vi "Write File Path.vi"(8 "error in (no error)":errorcluster, 10 "File Path":path, 11 "File Parser Interface in":refnum<class "File Parser Interface.lvclass">) -> (0 "error out":errorcluster, 3 "File Parser Interface out":refnum<class "File Parser Interface.lvclass">)   [LabVIEW 2018, in "File Parser Interface.lvlib" / "File Parser Interface.lvclass"]
uses:
  File Parser Interface.lvclass
  File Parser Interface.lvclass/File Parser Interface.ctl
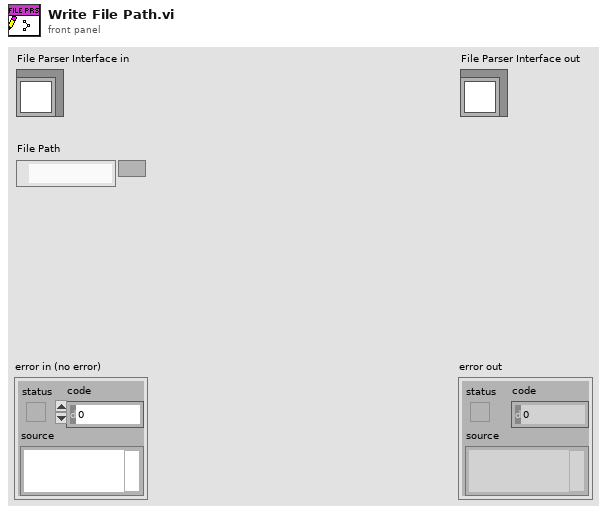
[diagram p1: front panel]
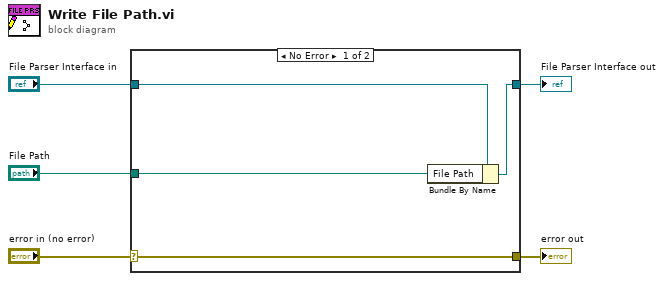
[diagram p0: block diagram]
diagram:
  n1 = case shown="No Error" "error in (no error)" {
    selector: "error in (no error)" -> [w9 w10]
    tunnel: [w9 w10] -> w4
    tunnel: [w7 w11] -> w2
    tunnel: "File Parser Interface in" -> [w8 w11]
    tunnel: "File Path" -> [w6 _]
    frame No Error {
      n2 = Bundle By Name(cluster=w8, "File Path"=w6) -> (w7:refnum<class "File Parser Interface.lvclass">)
    }
    frame Error {
    }
  }
  "error out" <- w4
  "File Parser Interface out" <- w2
